vi "FTW-Logger-Launch.vi"(5 "FTW Logger Configuration":string="{\n  \"Identity\": \"EventLog\",\n  \"InboxAddress\": \"tcp://127.0.0.1:*\",\n  \"PublisherAddress\": \"\",\n  \"DebugShowPanel\": false,\n  \"DebugEnableInboxLogging\": false,\n  \"DebugEnableJobLogging\": false,\n  \"ApplicationName\": \"Featherweight Application\",\n  \"LoggerName\": \"Log\",\n  \"LoggerDirectory\": \"[UserAppDir]\\\\Featherweight\\\\Logs\",\n  \"LoggerDiskThrashDelay\": 200\n}", 11 "error in":errorcluster) -> (4 "FTW Logger Connector":refnum<class "FTW-Logger.lvclass">, 6 "Logger Address":string, 15 "error out":errorcluster)   [LabVIEW 2013, in "FTW-Actor.lvlib" / "FTW-Logger.lvclass"]
doc: "This method launches a Logger Process which is then referred to based on its LoggerID. Normally in a LabVIEW application, an object's methods would adhere to dataflow with the object wired to the method; however, the Logger Process object likely needs to be accessed by many different portions of your application, and for this reason, it is called by reference, where the LoggerID string refers to the logger.\n\nThis method should be called as one of the very first actions in your application to reasonably ensure the buffer of logged events does not overflow. Events that are logged prior to launching the Logger Process with this method are queued, and will be logged once this process begins."
uses:
  FTW-Logger.lvclass
  Connector/FTW-ActorConnector.lvclass
  Core/FTW-Logger-Process.vi
  Core/FTW-Logger-Core.lvclass
panel:
  # "Inputs"
  # "Outputs"
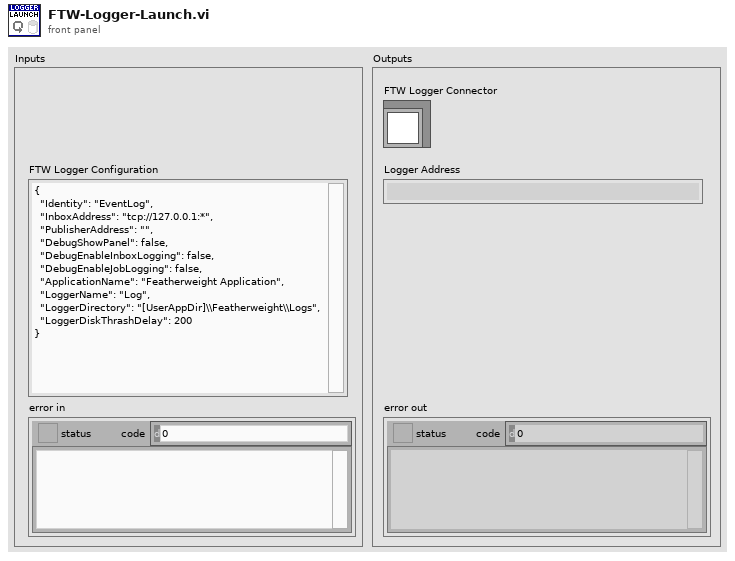
[diagram p1: front panel]
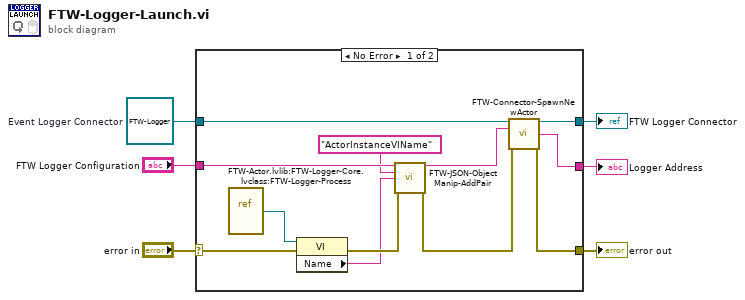
[diagram p0: block diagram]
diagram:
  w3 = refnum<class "FTW-Logger.lvclass"> refnum  # Event Logger Connector
  n1 = case shown="No Error" "error in" {
    selector: "error in" -> [w13 w20]
    tunnel: [w16 w20] -> w6
    tunnel: [w17 w19] -> w4
    tunnel: w3 -> [w18 w19]
    tunnel: "FTW Logger Configuration" -> [w12 _]
    tunnel: [w15 _] -> w1
    frame No Error {
      n2 = vi-ref "FTW-Actor.lvlib:FTW-Logger-Core.lvclass:FTW-Logger-Process.vi"() -> (w14:refnum<vi>)
      n3 = property class="VI"(reference=w14, error in=w13) -> (error out=w10:errorcluster, "Name"=w7:string)  [unwired: 1 out]
      n4 = call "FTW-JSON-ObjectManip-AddPair.vi"("Input JSON Object"=w12, "Key"="ActorInstanceVIName", "Value"=w7, "error in"=w10) -> ("Output JSON Object"=w11:string, "error out"=w9:errorcluster)  [unwired: 10 in]
      n5 = call "FTW-Connector-SpawnNewActor.vi"("FTW Actor Connector Type"=w18, "Instance Configuration"=w11, "error in"=w9) -> ("FTW Actor Connector"=w17:refnum<class "FTW-Logger.lvclass">, "Instance Inbox Address"=w15:string, "error out"=w16:errorcluster)  [unwired: 8 in, 2 out]
    }
    frame Error {
    }
  }
  "error out" <- w6
  "FTW Logger Connector" <- w4
  "Logger Address" <- w1
